vi "PlotData Data.vi"() -> (0 "Plot Data":T1 {"Configuration"."Sliders"."Instrument Sequence" scale=0.0..10.0; "Configuration"."Sliders"."Strain Sequence" scale=0.0..10.0})   [LabVIEW 2014]
uses:
  PlotData Data.ctl
  PlotData Config.ctl
  Measurement.ctl
  WhichInstrument.ctl
  Hardware Control/Parameter Analyzer/Electrical Data.ctl
  Hardware Control/Spectrometer/Spectral Data.ctl
  Instrument Sequence/Instrument Steps.ctl
  Instrument Sequence/Action.ctl
  Instrument Sequence/Instrument List.ctl
  PlotData Refnums.ctl
  Chooseplot.ctl
  Electrical Data Plot Refnums.ctl
  Optical Spectrum Plot Refnum.ctl
  PlotData Initialization.ctl
panel:
  # "LICENSED MATERIALS – PROPERTY OF IBM\nCopyright IBM Corp. 2016,\nALL RIGHTS RESERVED"
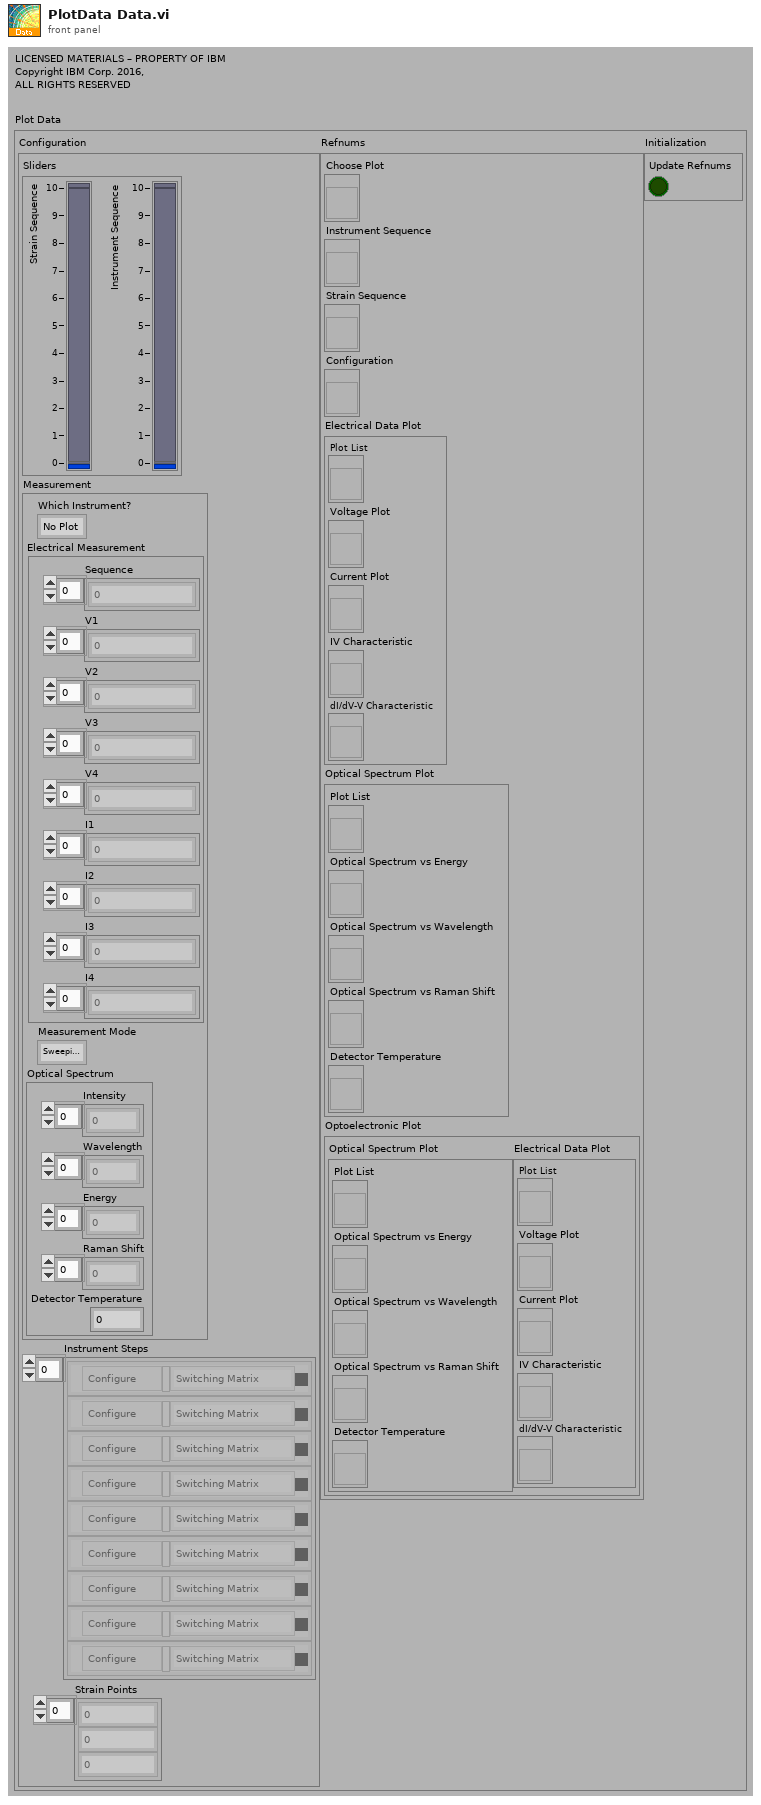
[diagram p1: front panel]
types:
  T1 = typedef "PlotData Data.ctl" = cluster{"Configuration":T2, "Refnums":T10, "Initialization":T13}
  T2 = typedef "PlotData Config.ctl" = cluster{"Sliders":cluster{"Strain Sequence":i32, "Instrument Sequence":i32}, "Measurement":T3, "Instrument Steps":T7, "Strain Points":dbl[]}
  T3 = typedef "Measurement.ctl" = cluster{"Which Instrument?":T4, "Electrical Measurement":T5, "Measurement Mode":enum16{"Sweeping Mode", "Sampling Mode"}, "Optical Spectrum":T6}
  T4 = typedef "WhichInstrument.ctl" = enum16{"No Plot", "Spectrometer", "Parameter Analyzer", "Optoelectronic"}
  T5 = typedef "Electrical Data.ctl" = cluster{"Sequence":dbl[], "V1":dbl[], "V2":dbl[], "V3":dbl[], "V4":dbl[], "I1":dbl[], "I2":dbl[], "I3":dbl[], "I4":dbl[]}
  T6 = typedef "Spectral Data.ctl" = cluster{"Intensity":dbl[], "Wavelength":dbl[], "Energy":dbl[], "Raman Shift":dbl[], "Detector Temperature":dbl}
  T7 = typedef "Instrument Steps.ctl" = cluster{"Action":T8, "Configuration":variant, "Instrument":T9, "Status":enum8{"False", "True", "Mixed"}}[]
  T8 = typedef "Action.ctl" = enum32{"Configure", "Measure"}
  T9 = typedef "Instrument List.ctl" = enum32{"Unknown Instrument", "Switching Matrix", "Parameter Analyzer", "Optical Spectrometer", "Optoelectronic", "Autofocus"}
  T10 = typedef "PlotData Refnums.ctl" = cluster{"Choose Plot":refnum<vi>, "Instrument Sequence":refnum<vi>, "Strain Sequence":refnum<vi>, "Configuration":refnum<vi>, "Electrical Data Plot":T11, "Optical Spectrum Plot":T12, "Optoelectronic Plot":cluster{"Optical Spectrum Plot":T12, "Electrical Data Plot":T11}}
  T11 = typedef "Electrical Data Plot Refnums.ctl" = cluster{"Plot List":refnum<vi>, "Voltage Plot":refnum<vi>, "Current Plot":refnum<vi>, "IV Characteristic":refnum<vi>, "dI/dV-V Characteristic":refnum<vi>}
  T12 = typedef "Optical Spectrum Plot Refnum.ctl" = cluster{"Plot List":refnum<vi>, "Optical Spectrum vs Energy":refnum<vi>, "Optical Spectrum vs Wavelength":refnum<vi>, "Optical Spectrum vs Raman Shift":refnum<vi>, "Detector Temperature":refnum<vi>}
  T13 = typedef "PlotData Initialization.ctl" = cluster{"Update Refnums":bool}
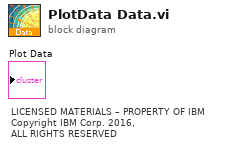
[diagram p0: block diagram]
diagram:
  # "LICENSED MATERIALS – PROPERTY OF IBM\nCopyright IBM Corp. 2016,\nALL RIGHTS RESERVED"
